vi "Receive_Packet.vi"(5 "Packet? (t)":bool=TRUE, 6 "clear_timeout_error (f)":bool, 7 "mode (standard)":T1(ring), 8 "error in (no error)":errorcluster, 10 "Offset (0)":u32=548, 11 "Socket.UDP in":refnum<class "Socket.UDP.lvclass">) -> (0 "error out":errorcluster, 1 "bytes_read":i32, 2 "data out":string, 3 "Socket.UDP out":refnum<class "Socket.UDP.lvclass">)   [LabVIEW 2014, in "Socket.lvlib" / "Socket.UDP.lvclass"]
doc: "enum mode ignored for UDP.\n\nI32 bufsize is the maximum number of bytes to read. Default is 548 and if you wire any value other than 548 to bufsize, windows mya return an error because the function cannot read fewer bytes than are in a packet\n\nbool clear_timeout_error optional input to clear the timeout error before exiting the method. This is used when looping receive to check for loop exit conditions."
uses:
  Socket.UDP.lvclass
  Socket.UDP.lvclass/Socket.UDP.ctl
  Socket.Base/Socket.Base.lvclass/Socket.Base.ctl
  Accessors/Read udp_refnum.vi
  Socket.Base/Accessors/Read timeout.vi
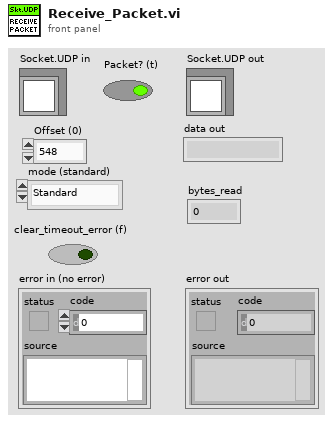
[diagram p1: front panel]
types:
  T1 = enum16{"Standard", "Buffered", "CRLF", "Immediate"}
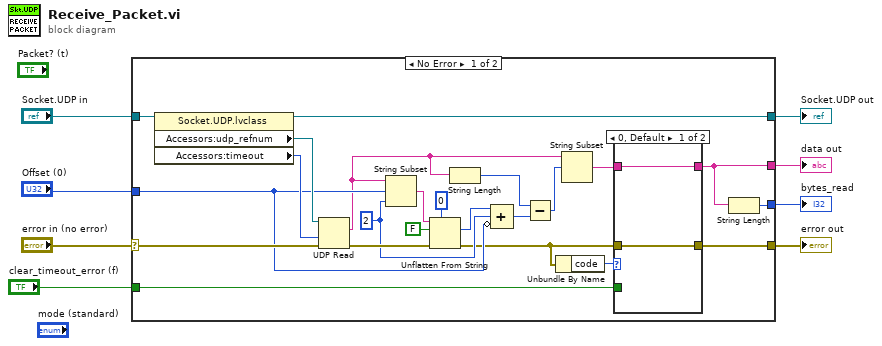
[diagram p0: block diagram]
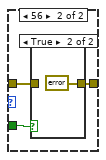
[diagram p2: hidden frame]
diagram:
  n1 = case shown="No Error" "error in (no error)" {
    selector: "error in (no error)" -> [w30 w40]
    tunnel: [w22 w40] -> w7
    tunnel: [w29 w39] -> w5
    tunnel: "Socket.UDP in" -> [w31 w39]
    tunnel: "Offset (0)" -> [w15 _]
    tunnel: [w26 _] -> w4
    tunnel: [w24 _] -> w3
    tunnel: "clear_timeout_error (f)" -> [w23 _]
    frame No Error {
      w16 = 2 ("length (rest)")
      n2 = property class="Socket.UDP.lvclass"(reference=w31) -> (reference out=w29:refnum<class "Socket.UDP.lvclass">, "Accessors:udp_refnum"=w28:refnum<k16>, "Accessors:timeout"=w27:i32)  [unwired: 1 in, 1 out]
      n3 = UDP Read(connection ID=w28, timeout ms (25000)=w27, 8:w30) -> (data out=w12:string, error out=w18:errorcluster)  [unwired: 1 in, 3 out]
      n4 = String Subset(string=w12, offset (0)=w15, length (rest)=w16) -> (substring=w19:string)
      n5 = Unflatten From String(type=u16 0, binary string=w19, data includes array or string size? (T)=FALSE, error in (no error)=w18) -> (value=w17:u16, error out=w14:errorcluster)  [unwired: 1 in, 1 out]
      n6 = String Length(string=w12) -> (length=w11:i32)
      n7 = Compound Arithmetic op=ADD(w17, w16, invert w15) -> (w13:u32)
      n8 = Subtract(x=w11, y=w13) -> (x-y=w10:u32)
      n9 = Unbundle By Name(w14) -> ("code"=w25:i32)
      n10 = String Subset(string=w12, offset (0)=w10) -> (substring=w9:string)  [unwired: 1 in]
      n11 = case shown="0, Default" w25 {
        tunnel: w14 -> [w33 w34]
        tunnel: w9 -> [w32 _]
        tunnel: [w33 w35] -> w22
        tunnel: [w32 _] -> w24
        tunnel: w23 -> [_ w36]
        frame 0, Default {
        }
        frame 56 {
          n12 = case shown="True" w36 {
            tunnel: [w37 errorcluster {"status"=FALSE, "code"=0, "source"=""} ("error constant")] -> w35
            tunnel: w34 -> [w37 _]
            frame False {
            }
            frame True {
            }
          }
        }
      }
      n13 = String Length(string=w24) -> (length=w26:i32)
    }
    frame Error {
    }
  }
  "error out" <- w7
  "Socket.UDP out" <- w5
  "data out" <- w3
  "bytes_read" <- w4
